vi "Serial.vi"(7 "States":T1, 8 "error in":errorcluster, 9 "Command":string="*IDN?", 10 "baud rate":u32=9600, 11 "Alias":string) -> (0 "error out":errorcluster, 3 "Output":string)   [LabVIEW 2021, in "Wrappers.lvlib"]
uses:
  Wrappers.lvlib
  Controls/Serial States.ctl
  Load INI/Controls/Instruments_Data.ctl
  63192432-051e-435b-80d3-99e6299f4ad3.vi
  <vilib>/Instr/_visa.llb/VISA Configure Serial Port (Instr).vi
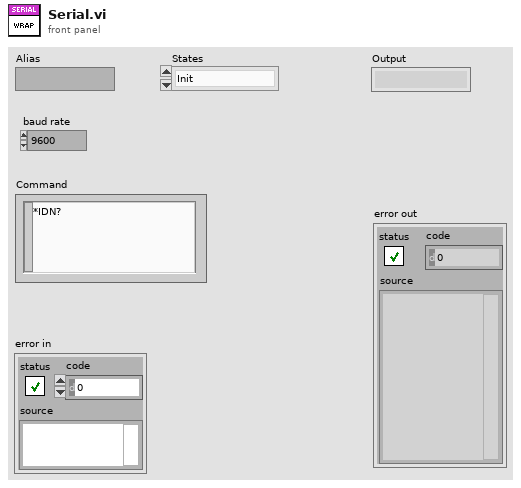
[diagram p1: front panel]
types:
  T1 = typedef "Wrappers.lvlib/Serial States.ctl" = enum16{"Init", "Read", "Write", "Close"}
  T2 = typedef "Instruments_Data.ctl" = cluster{"Alias":string, "Resource ":string}
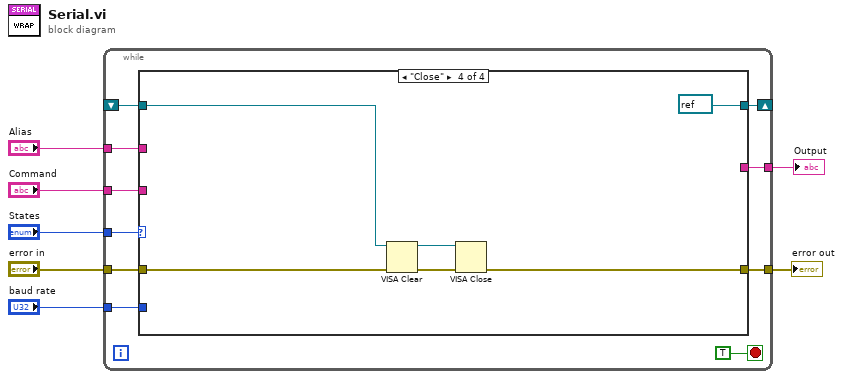
[diagram p0: block diagram]
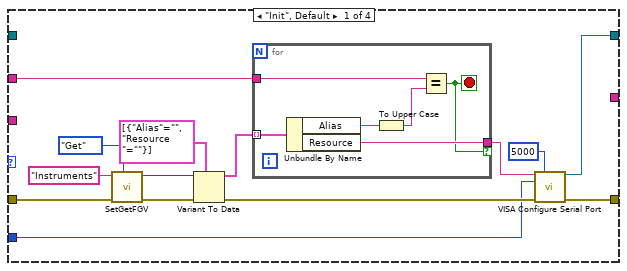
[diagram p2: hidden frame]
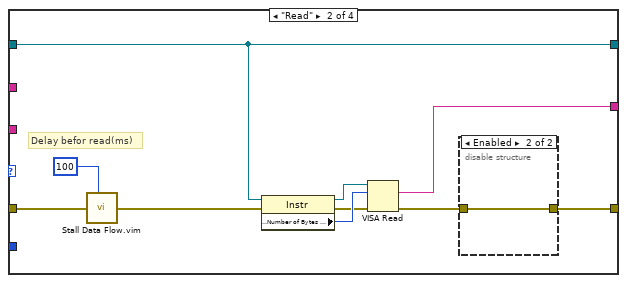
[diagram p3: hidden frame]
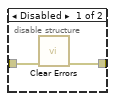
[diagram p4: hidden frame]
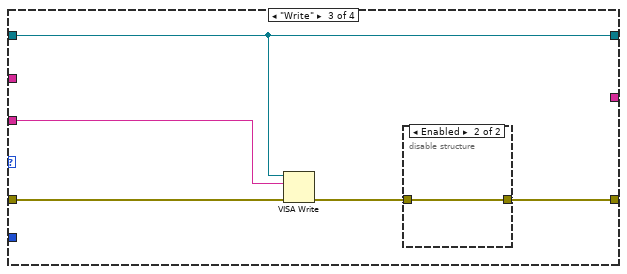
[diagram p5: hidden frame]
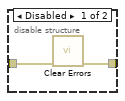
[diagram p6: hidden frame]
diagram:
  n1 = while {
    tunnel: "States" -> [w16]
    tunnel: "error in" -> [w15]
    tunnel: "baud rate" -> [w14]
    tunnel: "Alias" -> [w13]
    shift-right: [w12] -> _
    shift-left: _ -> [w11]
    tunnel: [w10] -> w3
    tunnel: [w9] -> w2
    tunnel: "Command" -> [w8]
    stop <- TRUE stop-if-true
    n2 = case shown="\"Close\"" w16 {
      tunnel: w15 -> [w27 w47 w55 w62]
      tunnel: w14 -> [w18 _ _ _]
      tunnel: w13 -> [w23 _ _ _]
      tunnel: [w21 w38 w53 refnum<visa-resource-name> refnum ("VISA resource name out")] -> w12
      tunnel: w11 -> [_ w38 w53 w60]
      tunnel: [w20 w39 w51 w61] -> w10
      tunnel: [_ w40 _ _] -> w9
      tunnel: w8 -> [_ _ w52 _]
      frame "Init", Default {
        n3 = call "SetGetFGV.vi"("Method (Get)"=enum16{"Get", "Set"}."Get", "error in"=w27, "FGVname"="Instruments" ("Name")) -> ("error out"=w29:errorcluster, "Data out"=w30:variant)  [unwired: 7 in]
        n4 = Variant To Data(error in=w29, type=T2[] [{"Alias"="", "Resource "=""}], Variant=w30) -> (data=w24:T2[], error out=w26:errorcluster)
        n5 = for {
          tunnel: w24 -> [w37] mode=indexing
          tunnel: w23 -> [w36]
          tunnel: [w33] -> w22 if=w32
          stop <- w32 stop-if-true
          n6 = Unbundle By Name(w37) -> ("Alias"=w34:string, "Resource"=w33:string)
          n7 = To Upper Case(1:w34) -> (0:w35:string)
          n8 = Equal?(x=w36, y=w35) -> (x = y?=w32:bool)
        }
        n9 = call-poly "VISA Configure Serial Port"("VISA resource name"=w22, "timeout (10sec)"=u32 5000, "baud rate (9600)"=w18, "error in (no error)"=w26) -> ("VISA resource name out"=w21:refnum<visa-resource-name>, "error out"=w20:errorcluster)  [unwired: 6 in, 4 out]
      }
      frame "Read" {
        # "Delay befor read(ms)"
        n10 = call "Stall Data Flow.vim"("value in"=w47, "milliseconds to wait"=u32 100) -> ("value out"=w42:errorcluster)  [unwired: 1 out]
        n11 = property class="Instr"(reference=w38, error in=w42) -> (reference out=w44:refnum<visa-resource-name>, error out=w43:errorcluster, "Serial Settings:Number of Bytes at Serial Port"=w45:u32)
        n12 = VISA Read(VISA resource name=w44, byte count=w45, error in (no error)=w43) -> (read buffer=w40:string, error out=w41:errorcluster)  [unwired: 2 out]
        n13 = disable-structure shown="Enabled" {
          disable-tunnel: w41 -> [w49 w50]
          disable-tunnel: [w48 w50] -> w39
          frame Disabled {
            n14 = call <vilib>:"Clear Errors.vi"("error in (no error)"=w49) -> ("error out"=w48:errorcluster)  [unwired: 5 in, 1 out]
          }
          frame Enabled {
          }
        }
      }
      frame "Write" {
        n15 = VISA Write(VISA resource name=w53, write buffer=w52, error in (no error)=w55) -> (error out=w54:errorcluster)  [unwired: 2 out]
        n16 = disable-structure shown="Enabled" {
          disable-tunnel: w54 -> [w57 w58]
          disable-tunnel: [w56 w58] -> w51
          frame Disabled {
            n17 = call <vilib>:"Clear Errors.vi"("error in (no error)"=w57) -> ("error out"=w56:errorcluster)  [unwired: 5 in, 1 out]
          }
          frame Enabled {
          }
        }
      }
      frame "Close" {
        n18 = VISA Clear(VISA resource name=w60, error in (no error)=w62) -> (VISA resource name out=w63:refnum<visa-resource-name>, error out=w64:errorcluster)
        n19 = VISA Close(VISA resource name=w63, error in (no error)=w64) -> (error out=w61:errorcluster)
      }
    }
  }
  "error out" <- w3
  "Output" <- w2
